vi "Stop.vi"(7 "Actor in":refnum<class "Actor.lvclass">, 8 "Error in":errorcluster) -> (5 "Actor out":refnum<class "Actor.lvclass">)   [LabVIEW 2025, in "jettl.lvlib" / "Actor.lvlib"]
uses:
  Actor.lvlib
  Actor/Actor.lvclass
  Teardown Location.ctl
  Stopped Msg/Tell Parent.vi
  Stopped Msg/Tell Child.vi
  Stopped Msg/Stopped Msg.lvlib
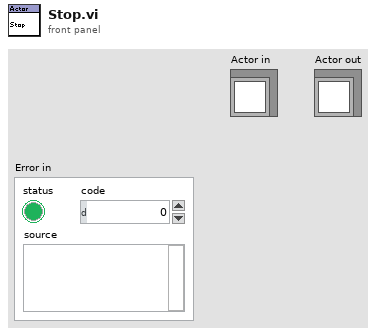
[diagram p1: front panel]
types:
  T1 = typedef "jettl.lvlib/Actor.lvlib/Teardown Location.ctl" = enum16{"Start", "Stop"}
  T2 = typedef "jettl.lvlib/Actor.lvlib/Child UIDs.ctl" = set{string}
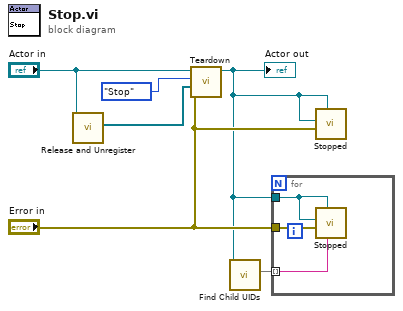
[diagram p0: block diagram]
diagram:
  n1 = call "Release and Unregister.vi"("Actor"="Actor in") -> ("Unhandled Msgs"=w5:refnum<class "Msg.lvclass">[])  [unwired: 10 in]
  n2 = call-dynamic "Teardown.vi"("Error in"="Error in", "Unhandled Msgs"=w5, "Teardown Location"=Teardown_Location."Stop", "Actor in"="Actor in") -> ("Actor out"=w1:refnum<class "Actor.lvclass">)  [unwired: 7 in]
  "Actor out" <- w1
  n3 = call-dynamic "Find Child UIDs.vi"("Actor in"=w1) -> ("Child UIDs"=w3:T2)  [unwired: 10 in]
  n4 = for {
    tunnel: w1 -> [w9]
    tunnel: w3 -> [w7] mode=indexing
    tunnel: "Error in" -> [w8]
    n5 = call-poly "Stopped.vi"("UID"=w7, "Actor in"=w9, "Error"=w8, "Actor"=w9) -> ()  [unwired: 7 in, 1 out]
  }
  n6 = call-poly "Stopped.vi"("Actor in"=w1, "Error"="Error in", "Actor"=w1) -> ()  [unwired: 8 in, 1 out]
